vi "Send Immediate Trigger.vi"(6 "Enable Channel 1 to 2":bool, 7 "Trigger Type (0: ARM)":i32(ring) items=["ARM", "Normal"], 8 "error in (no error)":errorcluster, 9 "Device Action (2: Both)":i32(ring)=2 items=["Acquire", "Transient", "Both"], 10 "Channel List ({Channel1})":i32[](array[ring])=[0] items=["Channel 1", "Channel 2"], 11 "VISA resource name":refnum<visa-resource-name>) -> (0 "error out":errorcluster, 3 "VISA resource name out":refnum<visa-resource-name>)   [LabVIEW 2026, in "Agilent B2900 Series.lvlib"]
doc: "Sends an arm trigger immediately for the specified device action to the specified channel. When the status of the specified device action is initiated, the arm trigger causes the layer change from arm to trigger."
uses:
  Agilent B2900 Series.lvlib
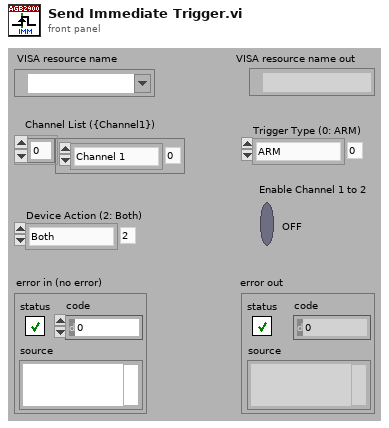
[diagram p1: front panel]
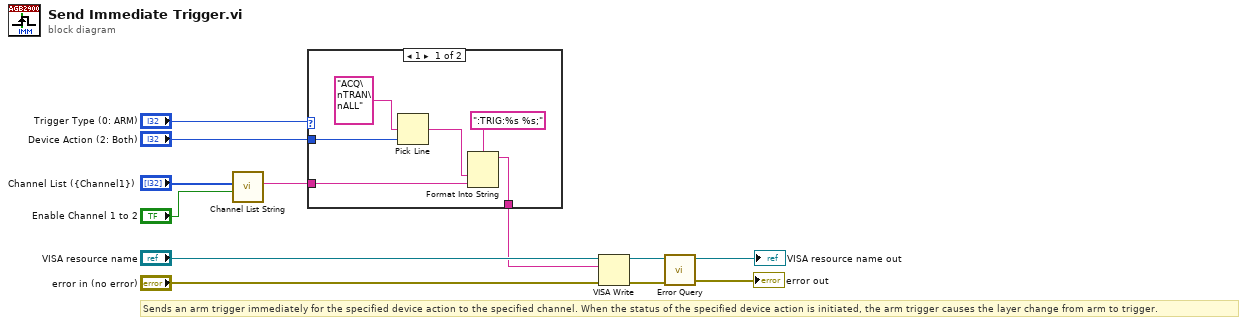
[diagram p0: block diagram]
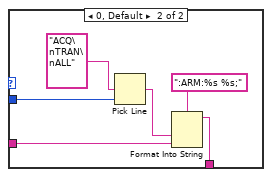
[diagram p2: hidden frame]
diagram:
  # "Sends an arm trigger immediately for the specified device action to the specified channel. When the status of the specified device action is initiated, the arm trigger causes the layer change from arm to trigger."
  n1 = call "Channel List String.vi"("Enable Channel 1 to 2"="Enable Channel 1 to 2", "Channel List ({Channel1})"="Channel List ({Channel1})") -> ("Channel List Command String"=w3:string)  [unwired: 9 in]
  n2 = case shown="1" "Trigger Type (0: ARM)" {
    tunnel: "Device Action (2: Both)" -> [w14 w23]
    tunnel: [w13 w21] -> w4
    tunnel: w3 -> [w16 w20]
    frame 1 {
      n3 = Pick Line(multi-line string="ACQ\nTRAN\nALL", line index=w14) -> (output string=w17:string)  [unwired: 1 in]
      n4 = Format Into String(format string=":TRIG:%s %s;", w17, w16) -> (resulting string=w13:string)  [unwired: 2 in, 1 out]
    }
    frame 0, Default {
      n5 = Pick Line(multi-line string="ACQ\nTRAN\nALL", line index=w23) -> (output string=w19:string)  [unwired: 1 in]
      n6 = Format Into String(format string=":ARM:%s %s;", w19, w20) -> (resulting string=w21:string)  [unwired: 2 in, 1 out]
    }
  }
  n7 = VISA Write(VISA resource name="VISA resource name", write buffer=w4, error in (no error)="error in (no error)") -> (VISA resource name out=w10:refnum<visa-resource-name>, error out=w9:errorcluster)  [unwired: 1 out]
  n8 = call "Error Query.vi"("error in (no error)"=w9, "VISA resource name"=w10) -> ("error out"=→"error out":errorcluster, "VISA resource name out"=→"VISA resource name out":refnum<visa-resource-name>)  [unwired: 6 in, 2 out]
